vi "DAC and ADC doesnt work.vi"() -> ()   [LabVIEW 2018]
uses:
  <vilib>/measure/NI_MABase.lvlib
  <vilib>/Waveform/WDTOps.llb/WDT Get XY Value DBL.vi
  <vilib>/Waveform/DWDTOps.llb/DWDT Analog to Digital.vi
panel:
  in  "stop":bool
  out "Analog reconstruction":waveform(dbl)(graph)
  out "Digital Sampling":digitalwaveform(graph)
  out "Analog":waveform(dbl)(graph)
  in  "amplitude":dbl=1.0 format="%0.2p"
  in  "frequency":dbl=10.0 format="%0.2p"
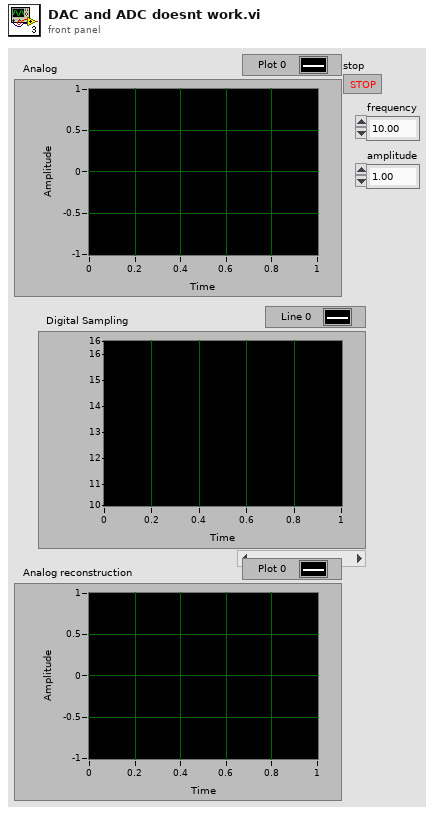
[diagram p1: front panel]
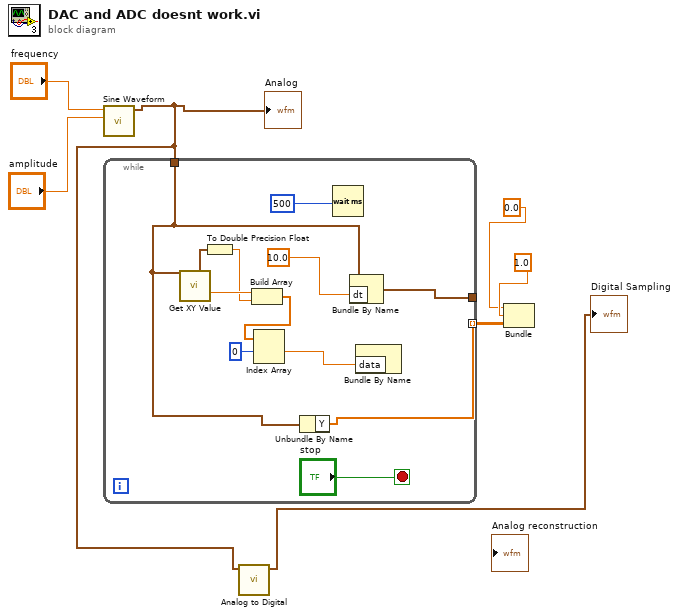
[diagram p0: block diagram]
diagram:
  n1 = call <vilib>:"Sine Waveform.vi"("amplitude"="amplitude", "frequency"="frequency") -> ("signal out"=w2:waveform(dbl))  [unwired: 8 in, 1 out]
  "Analog" <- w2
  n2 = while {
    tunnel: w2 -> [w12]
    tunnel: [w13] -> _
    tunnel: [w11] -> w5 mode=indexing
    stop <- "stop" stop-if-true
    n3 = call-poly <vilib>:"Get XY Value.vi"("Y position format"=w12) -> ("Y value"=w17:dbl, "X value"=w15:timestamp)  [unwired: 6 in, 3 out]
    n4 = To Double Precision Float(number=w15) -> (double precision float=w16:dbl)
    n5 = Build Array "Build Array"(w17, w16) -> (w10:dbl[])
    n6 = Index Array(array=w10, index #1=0 ("index")) -> (element #1=w9:dbl)  [unwired: 1 in, 1 out]
    n7 = Unbundle By Name(w12) -> ("Y"=w11:dbl[])
    n8 = Wait (ms)(milliseconds to wait=u32 500 ("millisecond timer value")) -> ()  [unwired: 1 out]
    n9 = Bundle By Name(cluster=w12, "dt"=10.0) -> (w13:waveform(dbl))
    n10 = Bundle By Name("data"=w9) -> ()  [unwired: 1 in, 1 out]
  }
  n11 = call-poly <vilib>:"Analog to Digital.vi"("analog waveform"=w2) -> ("digital waveform"=→"Digital Sampling":digitalwaveform)  [unwired: 7 in, 3 out]
  n12 = Bundle(0.0, 1.0, "Y"=w5) -> ()  [unwired: 1 in, 1 out]
